vi "MoAgSy_Agent_deinitialize_wrap.vi"(8 "error in (no error)":errorcluster, 11 "HGF_Agent in":refnum<class "MoAgSy_AgentBase.lvclass">) -> (0 "error out":errorcluster)   [LabVIEW 2009, in "MoAgSy_Base.lvlib" / "MoAgSy_AgentBase.lvclass"]
uses:
  MoAgSy_AgentBase.lvclass
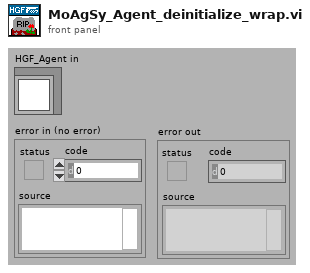
[diagram p1: front panel]
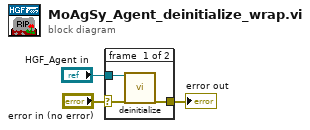
[diagram p0: block diagram]
diagram:
  n1 = case shown="No Error" "error in (no error)" {
    selector: "error in (no error)" -> [w6 w7]
    tunnel: [w5 w7] -> w2
    tunnel: "HGF_Agent in" -> [w4 _]
    frame #0 {
      n2 = call-dynamic "deinitialize.vi"("HGF_Agent"=w4, "error in (no error)"=w6) -> ("error out"=w5:errorcluster)  [unwired: 17 in]
    }
    frame #1 {
    }
  }
  "error out" <- w2
